vi "init runtime data structures.vi"(8 "error in":errorcluster, 9 "data allocations":T1, 10 "tag select":T4[](array[typedef]), 11 "tag select module runtime in":refnum<class "tag select module runtime.lvclass">) -> (0 "error out":errorcluster, 3 "tag select module runtime out":refnum<class "tag select module runtime.lvclass">)   [LabVIEW 2013, in "tag select module runtime.lvclass"]
uses:
  tag select module runtime.lvclass
  configuration/tag select configuration.ctl
  <vilib>/NI/Tag Bus Module Framework/channel/TBM channel.lvclass
  <vilib>/NI/Tag Bus/tag/Data Type.ctl
  <vilib>/NI/Tag Bus Module Framework/channel/data tables.ctl
  <vilib>/NI/Tag Bus/dictionary/data dictionary.lvclass
  <vilib>/NI/Tag Bus/dictionary table pair.ctl
  <vilib>/NI/Tag Bus/table/data table.ctl
  runtime tag select configuration.ctl
  <vilib>/NI/Tag Bus/tag/tag descriptor.lvclass/tag descriptor.ctl
  tag select module runtime.lvclass/tag select module runtime.ctl
  <vilib>/NI/Tag Bus/tag/read tag name.vi
  <vilib>/NI/Tag Bus/dictionary/locate tag.vi
  <vilib>/NI/Tag Bus/tag/tag descriptor.lvclass
  configuration/tag select module configuration.lvclass
  <vilib>/NI/Tag Bus/table/data table.lvlib
  <vilib>/NI/Tag Bus/tag bus.lvlib
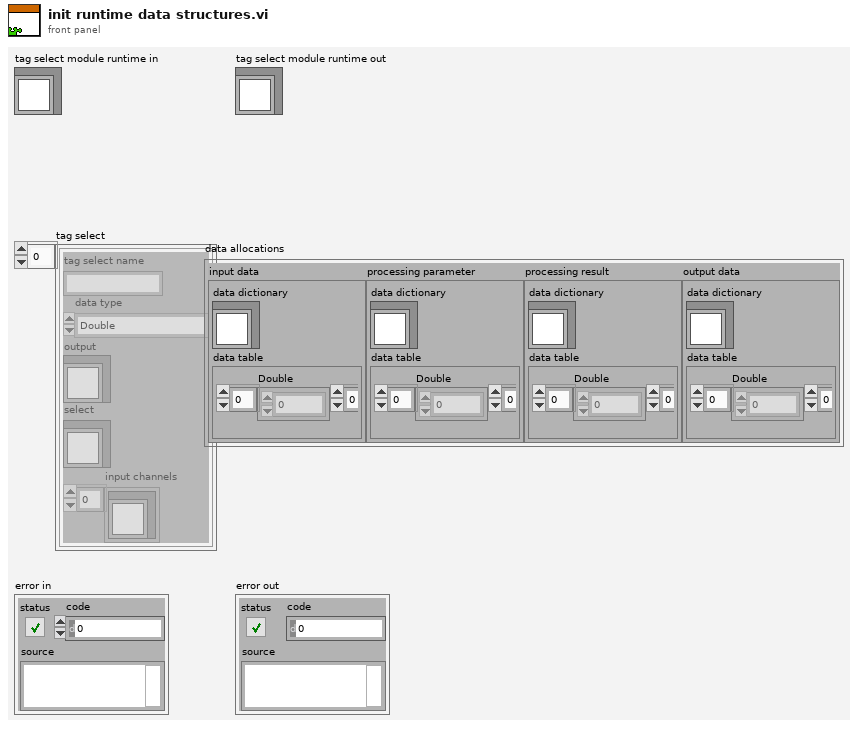
[diagram p1: front panel]
types:
  T1 = typedef "TBM channel.lvclass/data tables.ctl" = cluster{"input data":T2, "processing parameter":T2, "processing result":T2, "output data":T2}
  T2 = typedef "tag bus.lvlib/dictionary table pair.ctl" = cluster{"data dictionary":refnum<class "data dictionary.lvclass">, "data table":T3}
  T3 = typedef "tag bus.lvlib/data table.lvlib/data table.ctl" = cluster{"Double":dbl[], "Single":sgl[], "I64":i64[], "I32":i32[], "I16":i16[], "I8":i8[], "U64":u64[], "U32":u32[], "U16":u16[], "U8":u8[], "Boolean":bool[], "String":string[], "Array of Double":cluster{"DBL Array":dbl[]}[], "Array of Single":cluster{"SGL Array":sgl[]}[], "Array of I64":cluster{"I64 Array":i64[]}[], "Array of I32":cluster{"I32 Array":i32[]}[], "Array of I16":cluster{"I16 Array":i16[]}[], "Array of I8":cluster{"I8 Array":i8[]}[], "Array of U64":cluster{"U64 Array":u64[]}[], "Array of U32":cluster{"U32 Array":u32[]}[], "Array of U16":cluster{"U16 Array":u16[]}[], "Array of U8":cluster{"U8 Array":u8[]}[], "Array of Boolean":cluster{"Boolean Array":bool[]}[], "Array of String":cluster{"String Array":string[]}[]}
  T4 = typedef "tag select module configuration.lvclass/tag select configuration.ctl" = cluster{"tag select name":string, "data type":T5, "output":refnum<class "TBM channel.lvclass">, "select":refnum<class "TBM channel.lvclass">, "input channels":refnum<class "TBM channel.lvclass">[]}
  T5 = typedef "tag bus.lvlib/tag descriptor.lvclass/Data Type.ctl" = enum16{"Double", "Single", "I64", "I32", "I16", "I8", "U64", "U32", "U16", "U8", "Boolean", "String", "Array of Double", "Array of Single", "Array of I64", "Array of I32", "Array of I16", "Array of I8", "Array of U64", "Array of U32", "Array of U16", "Array of U8", "Array of Boolean", "Array of String"}
  T6 = typedef "runtime tag select configuration.ctl" = cluster{"output index":i32, "select index (bool)":i32, "input index":i32[], "data type":T5}
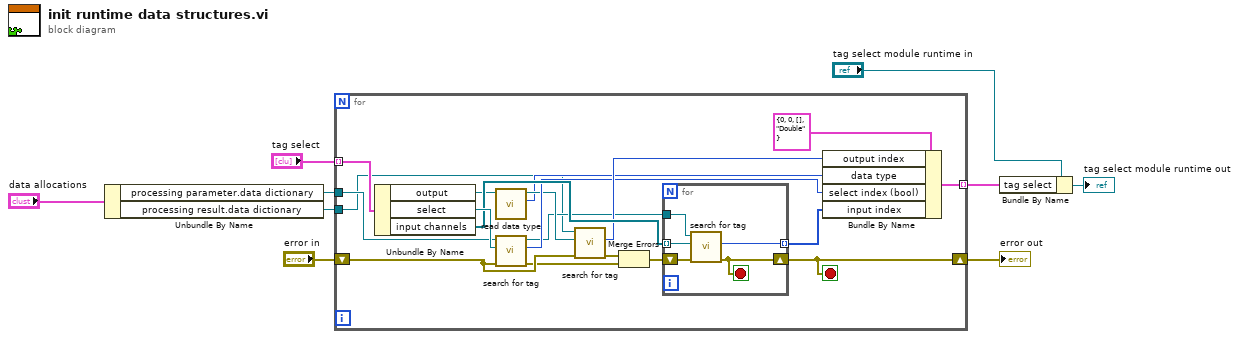
[diagram p0: block diagram]
diagram:
  n1 = Unbundle By Name("data allocations") -> ("processing parameter.data dictionary"=w2:refnum<class "data dictionary.lvclass">, "processing result.data dictionary"=w3:refnum<class "data dictionary.lvclass">)
  n2 = for {
    shift-right: [w25] -> w7
    shift-left: "error in" -> [w23]
    tunnel: "tag select" -> [w28] mode=indexing
    tunnel: [w26] -> w4 mode=indexing
    tunnel: w3 -> [w13]
    tunnel: w2 -> [w15]
    stop <- w25 stop-if-true
    n3 = Unbundle By Name(w28) -> ("output"=w18:refnum<class "TBM channel.lvclass">, "select"=w24:refnum<class "TBM channel.lvclass">, "input channels"=w22:refnum<class "TBM channel.lvclass">[])
    n4 = call <vilib>:"read data type.vi"("system tag in"=w18) -> ("data type"=w16:T5, "system tag out"=w17:refnum<class "TBM channel.lvclass">)  [unwired: 8 in, 1 out]
    n5 = call <vilib>:"search for tag.vi"("error in"=w23, "system tag"=w24, "data dictionary in"=w15) -> ("error out"=w12:errorcluster, "index"=w19:i32, "data dictionary out"=w14:refnum<class "data dictionary.lvclass">)  [unwired: 6 in]
    n6 = call <vilib>:"search for tag.vi"("error in"=w23, "system tag"=w17, "data dictionary in"=w13) -> ("error out"=w11:errorcluster, "index"=w20:i32)  [unwired: 6 in, 1 out]
    n7 = Merge Errors(w11, w12) -> (w10:errorcluster)
    n8 = for {
      shift-right: [w32] -> w25
      shift-left: w10 -> [w33]
      tunnel: w22 -> [w30] mode=indexing
      tunnel: [w31] -> w21 mode=indexing
      tunnel: w14 -> [w29]
      stop <- w32 stop-if-true
      n9 = call <vilib>:"search for tag.vi"("error in"=w33, "system tag"=w30, "data dictionary in"=w29) -> ("error out"=w32:errorcluster, "index"=w31:i32)  [unwired: 6 in, 1 out]
    }
    n10 = Bundle By Name(cluster=T6 {"output index"=0, "select index (bool)"=0, "input index"=[], "data type"=enum."Double"} ("alarm config"), "output index"=w20, "data type"=w16, "select index (bool)"=w19, "input index"=w21) -> (w26:T6)
  }
  "error out" <- w7
  n11 = Bundle By Name(cluster="tag select module runtime in", "tag select"=w4) -> (→"tag select module runtime out":refnum<class "tag select module runtime.lvclass">)
